vi "NXT arbiter A.vi"(0 "Tug array":i16[](array[numeric])=[0], 1 "Array angle\npointers":i16[](array[numeric])=[7, 8, 6, 9, 5, 10, 4, 11, 3, 12, 2, 13, 1, 14, 0, 15]) -> (2 "Arbiter Heading":i16, 3 "Arbiter\nvelocity":i16, 4 "Index":i16)   [LabVIEW 2012, in "ENGR3390 Tug Boat.lvrbt"]
doc: "This is the Mid Brain Arbiter. It accepts an array of I 16 each 16 long which is the sum of several behaviors. It calculates the location and value of the maximum point on the summed curve."
uses:
  <vilib>/NXT/Dual Mode Library/prims/sortArray/sortArray_int.vi
  ENGR3390 Tug Boat.lvrbt
panel:
  out "sorted array":i32[](array[numeric])
  out "Max value":i32
  out "Min value":i32
  out "Sum of all":cluster{i32, i32, "Tug array":i16[]}(graph)
  # "0"
  # "7"
  # "8"
  # "15"
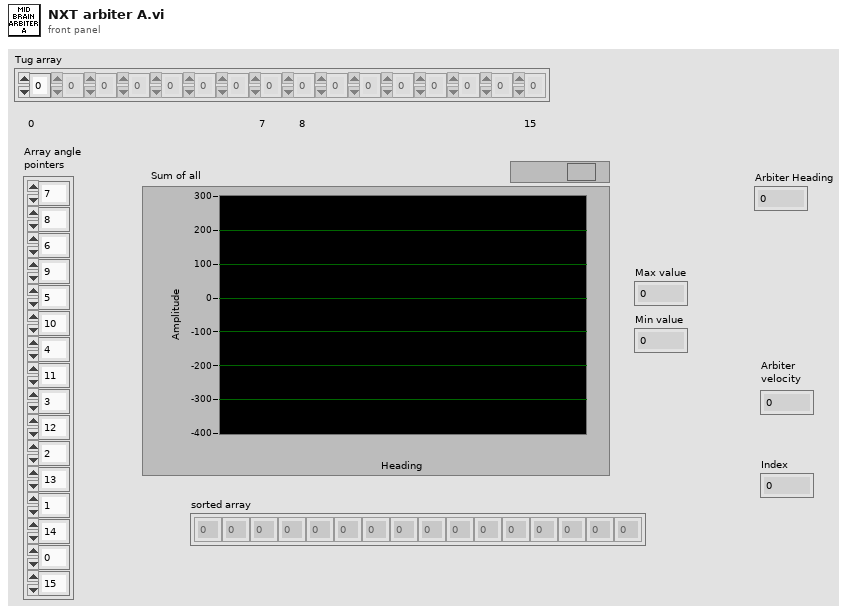
[diagram p1: front panel]
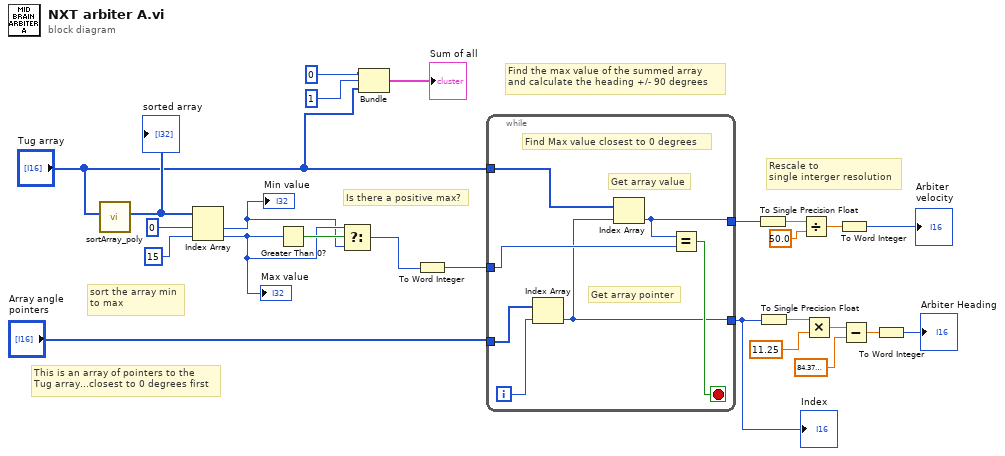
[diagram p0: block diagram]
diagram:
  # "Rescale to\nsingle interger resolution"
  # "This is an array of pointers to the\nTug array...closest to 0 degrees first"
  # "sort the array min\nto max"
  # "Is there a positive max?"
  # "Find the max value of the summed array\nand calculate the heading +/- 90 degrees"
  n1 = call-poly <vilib>:"sortArray_poly.vi"("array"="Tug array") -> ("sorted array"=w16:i32[])  [unwired: 10 in]
  "sorted array" <- w16
  n2 = Index Array(array=w16, index #1=0 ("index"), index #2=15 ("index")) -> (element #1=w9:i32, element #2=w10:i32)
  "Min value" <- w9
  "Max value" <- w10
  n3 = Greater Than 0?(x=w10) -> (x > 0?=w11:bool)
  n4 = Select(t=w10, s=w11, f=w9) -> (s? t:f=w8:i32)
  n5 = Bundle(0, 1, "Tug array"="Tug array") -> (→"Sum of all":cluster{i32, i32, "Tug array":i16[]})  [unwired: 1 in]
  n6 = To Word Integer(number=w8) -> (16bit integer=w12:i16)
  n7 = while {
    tunnel: w12 -> [w31]
    tunnel: "Tug array" -> [w32]
    tunnel: [w29] -> w5
    tunnel: "Array angle\npointers" -> [w27]
    tunnel: [w26] -> w6
    i -> [w28]
    stop <- w30 stop-if-true
    # "Get array value"
    # "Get array pointer"
    # "Find Max value closest to 0 degrees"
    n8 = Index Array(array=w27, index=w28) -> (element=w26:i16)
    n9 = Index Array(array=w32, index=w26) -> (element=w29:i16)
    n10 = Equal?(x=w29, y=w31) -> (x = y?=w30:bool)
  }
  "Index" <- w6
  n11 = To Single Precision Float(number=w5) -> (single precision float=w4:sgl)
  n12 = To Single Precision Float(number=w6) -> (single precision float=w17:sgl)
  n13 = Divide(x=w4, y=sgl 50.0) -> (x/y=w2:sgl)
  n14 = Multiply(x=w17, y=sgl 11.25) -> (x*y=w21:sgl)
  n15 = To Word Integer(number=w2) -> (16bit integer=→"Arbiter\nvelocity":i16)
  n16 = Subtract(x=w21, y=sgl 84.38) -> (x-y=w19:sgl)
  n17 = To Word Integer(number=w19) -> (16bit integer=→"Arbiter Heading":i16)
